vi "new현재시간(SubVI).vi"() -> (0 "시간 숫자":i32, 1 "시간 문자열":string, 2 "분":i32, 3 "시":i32, 4 "분 문자열":string, 5 "날짜/시간 문자열":string, 6 "시 문자열":string, 8 "초":i32, 9 "초 문자열":string)   [LabVIEW 2014]
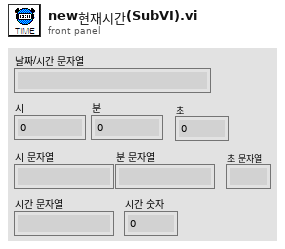
[diagram p1: front panel]
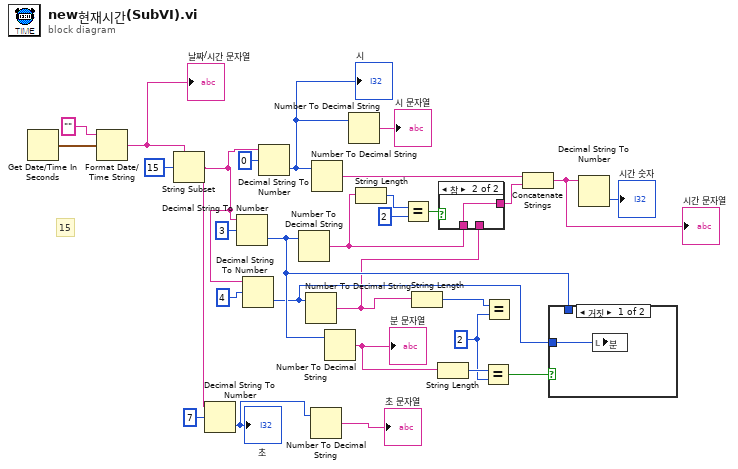
[diagram p0: block diagram]
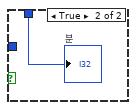
[diagram p3: hidden frame]
diagram:
  w11 = 2 ("y")
  # "15"
  n1 = Get Date/Time In Seconds() -> (seconds since 1Jan1904=w25:timestamp)
  n2 = Format Date/Time String(time format string (%c)="" ("시간 포맷 문자열 (%c)"), seconds (now)=w25) -> (date/time string=w16:string)  [unwired: 1 in]
  "날짜/시간 문자열" <- w16
  n3 = String Subset(string=w16, offset (0)=15 ("오프셋(0)")) -> (substring=w14:string)  [unwired: 1 in]
  n4 = Decimal String To Number(string=w14, offset=7 ("오프셋")) -> (number=w18:i32)  [unwired: 1 in, 1 out]
  "초" <- w18
  n5 = Decimal String To Number(string=w14, offset=3 ("오프셋")) -> (number=w8:i32)  [unwired: 1 in, 1 out]
  n6 = Decimal String To Number(string=w14, offset=4 ("오프셋")) -> (number=w7:i32)  [unwired: 1 in, 1 out]
  n7 = Decimal String To Number(string=w14, offset=0 ("오프셋")) -> (number=w21:i32)  [unwired: 1 in, 1 out]
  "시" <- w21
  n8 = Number To Decimal String(number=w8) -> (decimal integer string=w3:string)  [unwired: 1 in]
  n9 = Number To Decimal String(number=w7) -> (decimal integer string=w2:string)  [unwired: 1 in]
  n10 = Number To Decimal String(number=w18) -> (decimal integer string=→"초 문자열":string)  [unwired: 1 in]
  n11 = Number To Decimal String(number=w21) -> (decimal integer string=w29:string)  [unwired: 1 in]
  n12 = Number To Decimal String(number=w8) -> (decimal integer string=w10:string)  [unwired: 1 in]
  "분 문자열" <- w10
  n13 = Number To Decimal String(number=w21) -> (decimal integer string=→"시 문자열":string)  [unwired: 1 in]
  n14 = String Length(string=w3) -> (length=w6:i32)
  n15 = Equal?(x=w6, y=2) -> (x = y?=w4:bool)
  n16 = String Length(string=w2) -> (length=w13:i32)
  n17 = String Length(string=w10) -> (length=w12:i32)
  n18 = case shown="참" w4 {
    tunnel: w3 -> [_ w31]
    tunnel: w2 -> [w30 _]
    tunnel: [w30 w31] -> w1
    frame False {
    }
    frame True {
    }
  }
  n19 = Equal?(x=w12, y=w11) -> (x = y?=w9:bool)
  n20 = Equal?(x=w13, y=w11) -> ()  [unwired: 1 out]
  n21 = Concatenate Strings(w29, w1) -> (w23:string)
  "시간 문자열" <- w23
  n22 = case shown="거짓" w9 {
    tunnel: w8 -> [_ w33]
    tunnel: w7 -> [w32 _]
    frame False {
      n23 = local write "분"(w32) -> ()
    }
    frame True {
      "분" <- w33
    }
  }
  n24 = Decimal String To Number(string=w23) -> (number=→"시간 숫자":i32)  [unwired: 2 in, 1 out]
